vi "Find choosen target.vi"(10 "Map dimensions":dbl[](array[numeric]), 11 "Display map":u16[][](array[ring])) -> (2 "Numeric":dbl, 3 "Target location":dbl[](array[numeric]))   [LabVIEW 2015]
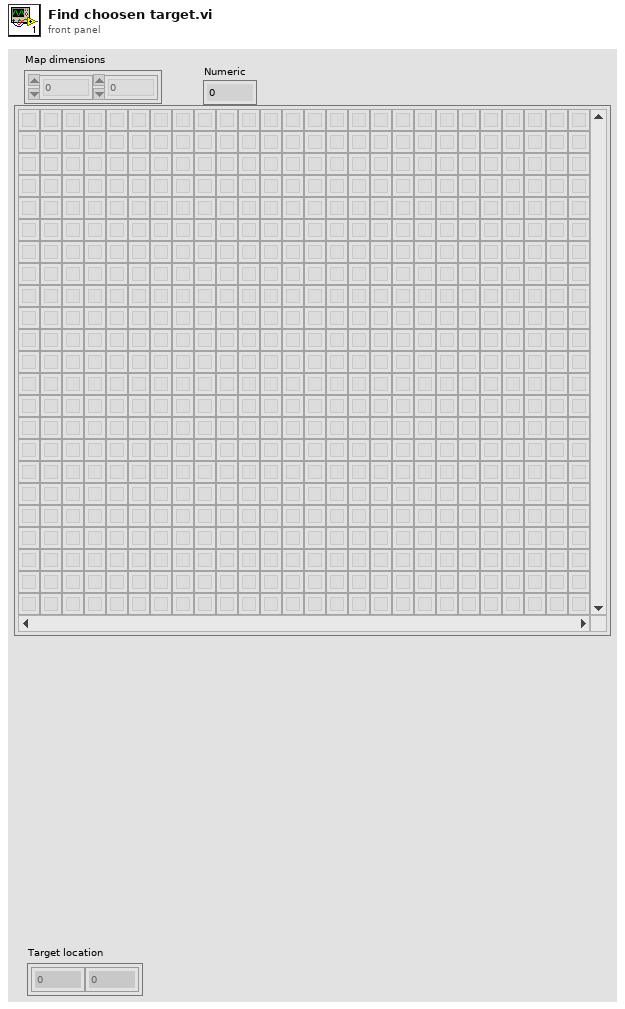
[diagram p1: front panel]
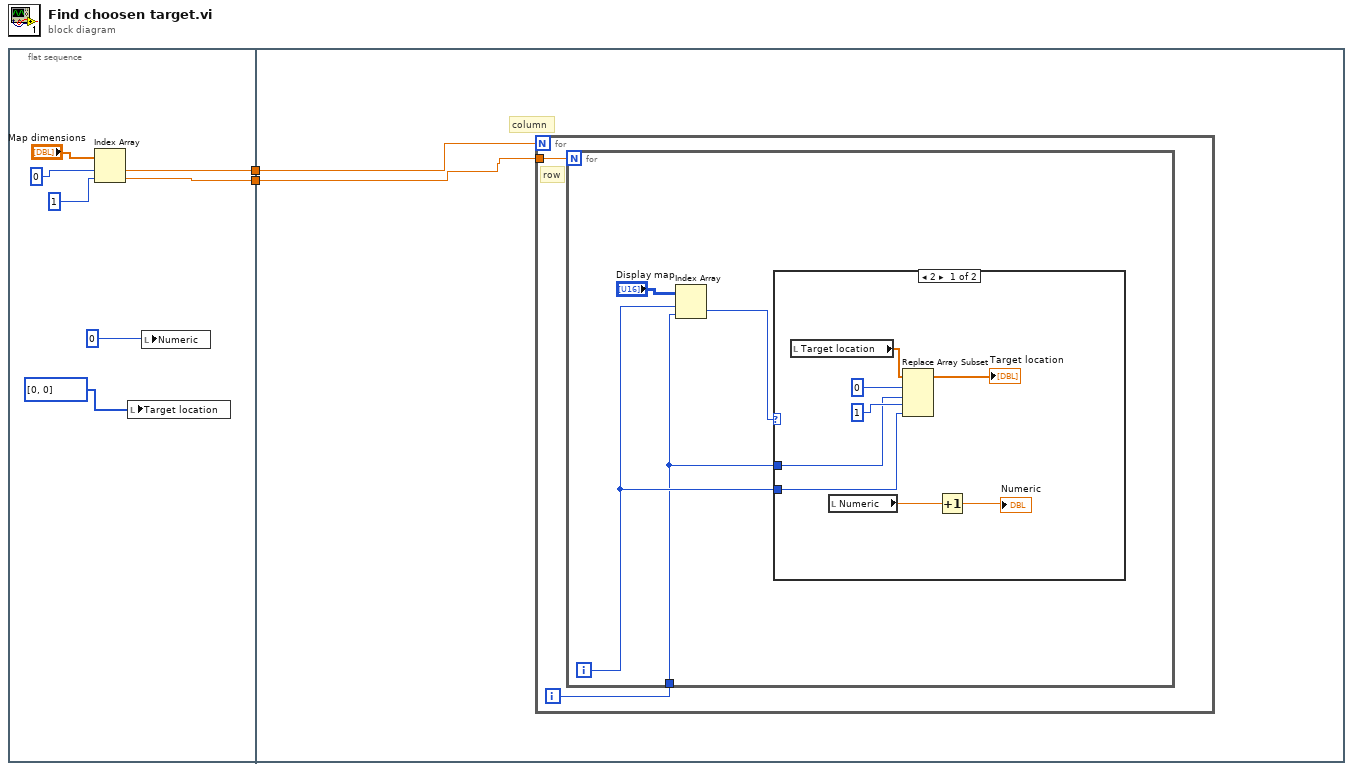
[diagram p0: block diagram]
diagram:
  n1 = flat-sequence {
    tunnel: [w6] -> w2
    tunnel: [w5] -> w1
    tunnel: w2 -> [w11]
    tunnel: w1 -> [w10]
    frame #0 {
      n2 = Index Array(array="Map dimensions", index #1=0, index #2=1) -> (element #1=w6:dbl, element #2=w5:dbl)
      n3 = local write "Target location"(i32[] [0, 0]) -> ()
      n4 = local write "Numeric"(0) -> ()
    }
    frame #1 {
      # "column"
      n5 = for {
        N: w11 -> [_]
        tunnel: w10 -> [w13]
        i -> [w12]
        # "row"
        n6 = for {
          N: w13 -> [_]
          tunnel: w12 -> [w14]
          i -> [w15]
          n7 = Index Array(array="Display map", index (row)=w15, index (col)=w14) -> (element=w16:u16)
          n8 = case shown="2" w16 {
            tunnel: w15 -> [w18 _]
            tunnel: w14 -> [w19 _]
            frame 2 {
              n9 = local read "Target location"() -> (w25:dbl[])
              n10 = local read "Numeric"() -> (w23:dbl)
              n11 = Replace Array Subset(array=w25, new element #1=w19, index #1=0, new element #2=w18, index #2=1) -> (→"Target location":dbl[])
              n12 = Increment(x=w23) -> (x+1=→"Numeric":dbl)
            }
            frame 1, Default {
            }
          }
        }
      }
    }
  }
